vi "[del]ZCAN_InitCAN( CANET ).vi"(4 "error in (no error)":errorcluster caption="错误输入（无错误）", 5 "ZCAN_InitCAN_setting_CANET":T1, 6 "device_hande":u32, 7 "设备类型":u32) -> (0 "error out":errorcluster caption="错误输出", 2 "can_index_handle":u32)   [LabVIEW 2011]
doc: "用于设置CAN通道的初始化参数。\n\n适用的设备：CANET-TCP ,CANET-UDP"
uses:
  data_type/ZCAN_InitCAN_setting_CANET.ctl
  bin/zlgcan_wrap.dll
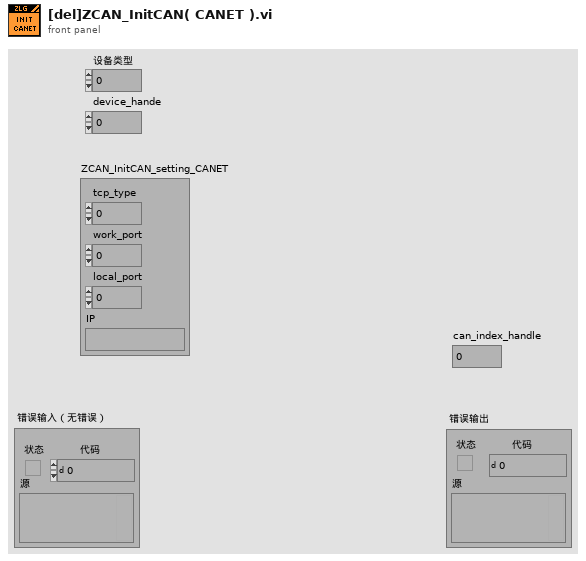
[diagram p1: front panel]
types:
  T1 = typedef "ZCAN_InitCAN_setting_CANET.ctl" = cluster{"tcp_type":u32, "work_port":u32, "local_port":u32, "IP":string}
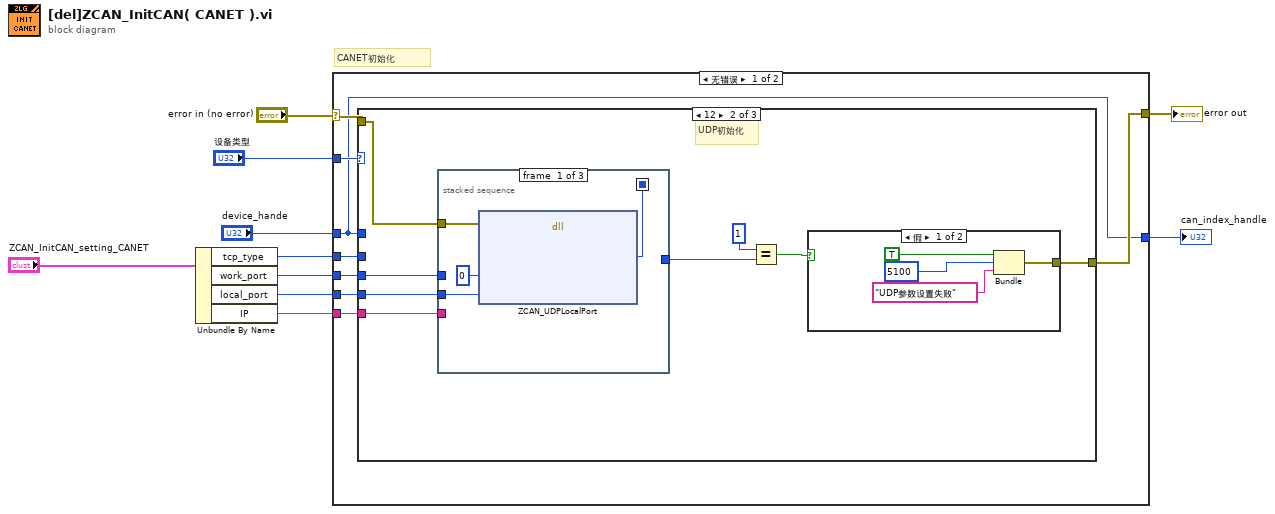
[diagram p0: block diagram]
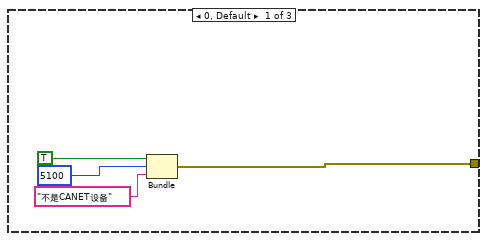
[diagram p2: hidden frame]
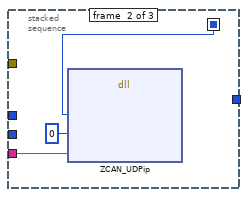
[diagram p3: hidden frame]
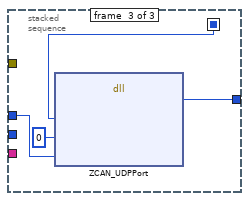
[diagram p4: hidden frame]
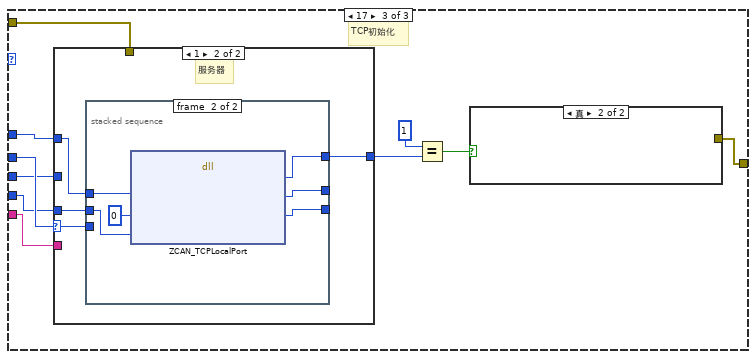
[diagram p6: hidden frame]
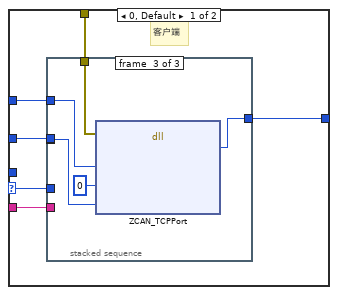
[diagram p7: hidden frame]
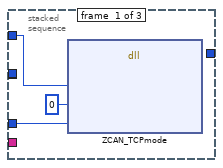
[diagram p8: hidden frame]
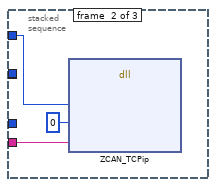
[diagram p9: hidden frame]
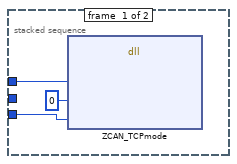
[diagram p10: hidden frame]
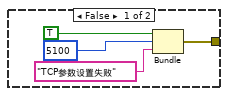
[diagram p11: hidden frame]
diagram:
  # "CANET初始化"
  n1 = Unbundle By Name("ZCAN_InitCAN_setting_CANET") -> ("tcp_type"=w8:u32, "work_port"=w6:u32, "local_port"=w5:u32, "IP"=w7:string)
  n2 = case shown="无错误" "error in (no error)" {
    selector: "error in (no error)" -> [w13 w91]
    tunnel: [w18 w91] -> w3
    tunnel: "设备类型" -> [w12 _]
    tunnel: "device_hande" -> [w11 w90]
    tunnel: w8 -> [w17 _]
    tunnel: w7 -> [w16 _]
    tunnel: w6 -> [w15 _]
    tunnel: w5 -> [w14 _]
    tunnel: [w11 w90] -> w4
    frame No Error {
      n3 = case "条件结构" shown="12" w12 {
        tunnel: [w19 w30 w47] -> w18
        tunnel: w11 -> [_ _ w52]
        tunnel: w17 -> [_ _ w51]
        tunnel: w16 -> [_ w28 w50]
        tunnel: w15 -> [_ w27 w49]
        tunnel: w14 -> [_ w29 w46]
        tunnel: w13 -> [_ w23 w48]
        frame 0, Default {
          n4 = Bundle("status"=TRUE, "code"=5100, "消息"="不是CANET设备") -> (w19:cluster{"status":bool, "code":i32, "消息":string})  [unwired: 1 in]
        }
        frame 12 {
          # "UDP初始化"
          n5 = stacked-sequence {
            seq-local: [w31 _ _] -> [_ w35 w38]
            tunnel: w29 -> [w33 _ _]
            tunnel: w28 -> [_ w37 _]
            tunnel: w27 -> [_ _ w41]
            tunnel: [_ _ w39] -> w24
            tunnel: w23 -> [w32 _ _]
            frame #0 {
              n6 = dll-call lib="C:/Users/binck/Desktop/[CODE]USBCAN/CANFD Tool/bin/zlgcan_wrap.dll" fn="ZCAN_UDPLocalPort"(error in=w32, "can_index"=u32 0, "local_port"=w33) -> ("hDev"=w31:u32)  [unwired: 6 in, 2 out]
            }
            frame #1 {
              n7 = dll-call lib="C:/Users/binck/Desktop/[CODE]USBCAN/CANFD Tool/bin/zlgcan_wrap.dll" fn="ZCAN_UDPip"("device_handle"=w35, "can_index"=u32 0, "ip"=w37) -> ()  [unwired: 7 in, 2 out]
            }
            frame #2 {
              n8 = dll-call lib="C:/Users/binck/Desktop/[CODE]USBCAN/CANFD Tool/bin/zlgcan_wrap.dll" fn="ZCAN_UDPPort"("hDev"=w38, "can_index"=u32 0, "work_port"=w41) -> ("return"=w39:u32)  [unwired: 6 in, 2 out]
            }
          }
          n9 = Equal?(x=1, y=w24) -> (x = y?=w25:bool)
          n10 = case shown="假" w25 {
            tunnel: [w42 _] -> w30
            frame False {
              n11 = Bundle("status"=TRUE, "code"=5100, "消息"="UDP参数设置失败") -> (w42:cluster{"status":bool, "code":i32, "消息":string})  [unwired: 1 in]
            }
            frame True {
            }
          }
        }
        frame 17 {
          # "TCP初始化"
          n12 = case shown="1" w51 {
            selector: w51 -> [w61 w76]
            tunnel: [w60 w75] -> w54
            tunnel: w52 -> [w59 w74]
            tunnel: w50 -> [w58 _]
            tunnel: w49 -> [w57 _]
            tunnel: w48 -> [w56 _]
            tunnel: w46 -> [_ w73]
            frame 0, Default {
              # "客户端"
              n13 = stacked-sequence {
                tunnel: w61 -> [w64 _ _]
                tunnel: [_ _ w72] -> w60
                tunnel: w59 -> [w62 w65 w71]
                tunnel: w58 -> [_ w66 _]
                tunnel: [_ _ w69] -> _
                tunnel: w57 -> [_ _ w69]
                tunnel: w56 -> [_ _ w68]
                frame #0 {
                  n14 = dll-call lib="C:/Users/binck/Desktop/[CODE]USBCAN/CANFD Tool/bin/zlgcan_wrap.dll" fn="ZCAN_TCPmode"("hDev"=w62, "can_index"=u32 0, "tcp_type"=w64) -> ()  [unwired: 7 in, 2 out]
                }
                frame #1 {
                  n15 = dll-call lib="C:/Users/binck/Desktop/[CODE]USBCAN/CANFD Tool/bin/zlgcan_wrap.dll" fn="ZCAN_TCPip"("device_handle"=w65, "can_index"=u32 0, "ip"=w66) -> ()  [unwired: 7 in, 2 out]
                }
                frame #2 {
                  n16 = dll-call lib="C:/Users/binck/Desktop/[CODE]USBCAN/CANFD Tool/bin/zlgcan_wrap.dll" fn="ZCAN_TCPPort"(error in=w68, "hDev"=w71, "can_index"=u32 0, "work_port"=w69) -> ("return"=w72:u32)  [unwired: 5 in, 2 out]
                }
              }
            }
            frame 1 {
              # "服务器"
              n17 = stacked-sequence {
                tunnel: w76 -> [w79 _]
                tunnel: [_ w85] -> w75
                tunnel: [_ w84] -> _
                tunnel: [_ w83] -> _
                tunnel: w74 -> [w77 w81]
                tunnel: w73 -> [_ w82]
                frame #0 {
                  n18 = dll-call lib="C:/Users/binck/Desktop/[CODE]USBCAN/CANFD Tool/bin/zlgcan_wrap.dll" fn="ZCAN_TCPmode"("hDev"=w77, "can_index"=u32 0, "tcp_type"=w79) -> ()  [unwired: 7 in, 2 out]
                }
                frame #1 {
                  n19 = dll-call lib="C:/Users/binck/Desktop/[CODE]USBCAN/CANFD Tool/bin/zlgcan_wrap.dll" fn="ZCAN_TCPLocalPort"("device_handle"=w81, "can_index"=u32 0, "local_port"=w82) -> ("return"=w85:u32, "device_handle"=w84:u32, "can_index"=w83:u32)  [unwired: 4 in, 2 out]
                }
              }
            }
          }
          n20 = Equal?(x=1, y=w54) -> (x = y?=w53:bool)
          n21 = case shown="真" w53 {
            tunnel: [w86 _] -> w47
            frame False {
              n22 = Bundle("status"=TRUE, "code"=5100, "消息"="TCP参数设置失败") -> (w86:cluster{"status":bool, "code":i32, "消息":string})  [unwired: 1 in]
            }
            frame True {
            }
          }
        }
      }
    }
    frame Error {
    }
  }
  "error out" <- w3
  "can_index_handle" <- w4
